vi "TagNormalizaction.vi"(6 "Inicio pasada":timestamp, 9 "Tiempo de paso (s)":dbl, 10 "TagData in":cluster{"TagCode":string, "FirstSeemUs":u64}[](array[cluster]), 11 "Tabla_flota":string[][](array[string])) -> (3 "Normalized Tags":string[](array[string]))   [LabVIEW 2015]
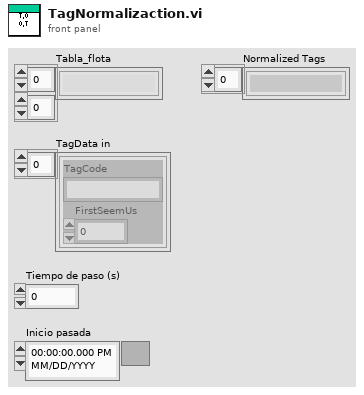
[diagram p1: front panel]
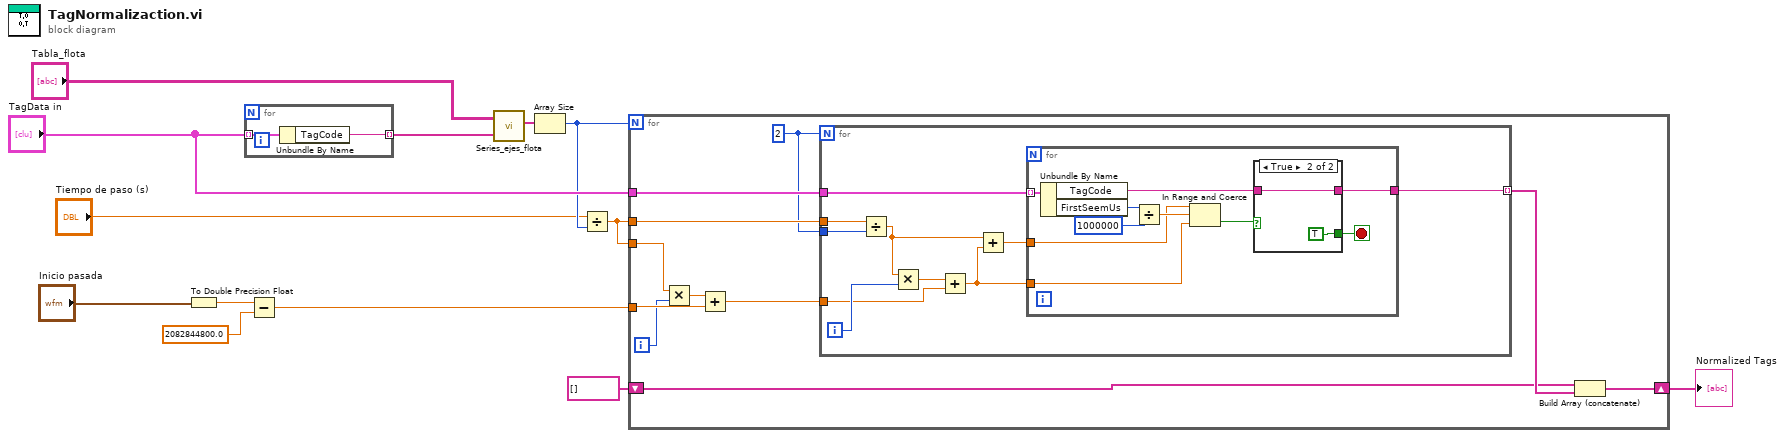
[diagram p0: block diagram]
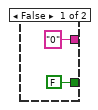
[diagram p2: hidden frame]
diagram:
  n1 = To Double Precision Float(number="Inicio pasada") -> (double precision float=w3:dbl)
  n2 = for {
    tunnel: "TagData in" -> [w15] mode=indexing
    tunnel: [w14] -> w7 mode=indexing
    n3 = Unbundle By Name(w15) -> ("TagCode"=w14:string)
  }
  n4 = Subtract(x=w3, y=2082844800.0) -> (x-y=w2:dbl)
  n5 = call "Series_ejes_flota.vi"("Tabla_flota"="Tabla_flota", "Tags"=w7) -> ("Series del convoy"=w6:string[])  [unwired: 2 in, 2 out]
  n6 = Array Size(array=w6) -> (size(s)=w9:i32)
  n7 = Divide(x="Tiempo de paso (s)", y=w9) -> (x/y=w11:dbl)
  n8 = for {
    N: w9 -> [_]
    tunnel: w2 -> [w25]
    tunnel: w11 -> [w16]
    tunnel: "TagData in" -> [w23]
    tunnel: w11 -> [w21]
    shift-right: [w18] -> w13
    shift-left: string[] [] -> [w17]
    i -> [w24]
    w20 = 2
    n9 = Multiply(x=w16, y=w24) -> (x*y=w26:dbl)
    n10 = Add(x=w26, y=w25) -> (x+y=w22:dbl)
    n11 = for {
      N: w20 -> [_]
      tunnel: w23 -> [w36]
      tunnel: w22 -> [w31]
      tunnel: w21 -> [w35]
      tunnel: w20 -> [w34]
      tunnel: [w27] -> w19 mode=indexing
      i -> [w33]
      n12 = Divide(x=w35, y=w34) -> (x/y=w29:dbl)
      n13 = Multiply(x=w29, y=w33) -> (x*y=w32:dbl)
      n14 = Add(x=w32, y=w31) -> (x+y=w30:dbl)
      n15 = Add(x=w29, y=w30) -> (x+y=w28:dbl)
      n16 = for {
        tunnel: w36 -> [w46] mode=indexing
        tunnel: w30 -> [w42]
        tunnel: w28 -> [w41]
        tunnel: [w38] -> w27
        stop <- w37 stop-if-true
        n17 = Unbundle By Name(w46) -> ("TagCode"=w39:string, "FirstSeemUs"=w45:u64)
        n18 = Divide(x=w45, y=u64 1000000) -> (x/y=w43:dbl)
        n19 = In Range and Coerce(upper limit=w41, x=w43, lower limit=w42) -> (In Range?=w40:bool)  [unwired: 1 out]
        n20 = case shown="True" w40 {
          tunnel: w39 -> [_ w50]
          tunnel: ["0" ("TagCode") w50] -> w38
          tunnel: [FALSE TRUE] -> w37
          frame False {
          }
          frame True {
          }
        }
      }
    }
    n21 = Build Array (concatenate)(w17, w19) -> (w18:string[])
  }
  "Normalized Tags" <- w13
